vi "4155C Config QSCV var1 params.vi"(4 "Cap Step":dbl=0.1 min=0.0 max=10.0 format="%.2f", 5 "compliance":dbl=0.1 min=0.0 max=0.1 format="%^.2e", 6 "step":dbl=2.0 min=-100.0 max=100.0 format="%^.4e", 7 "sweep mode":u16(ring) items=["Single", "Double"], 8 "error in (no error)":errorcluster, 9 "stop":dbl=1.0 min=-100.0 max=100.0 format="%^.4e", 10 "start":dbl min=-100.0 max=100.0 format="%^.4e", 11 "VISA session":refnum<visa-resource-name>) -> (0 "error out":errorcluster, 2 "Number of points":i32=1, 3 "dup VISA resource name":refnum<visa-resource-name>)   [LabVIEW 2016]
doc: "This VI configures the primary sweep source (VAR1) for a sweep mode measurement. \n* This VI does not perform error checking on MEASUREMENT MODE or UNIT TYPE of VAR1, therefore it is the application programmer's responsibility to make certain this VI is used in the proper mode."
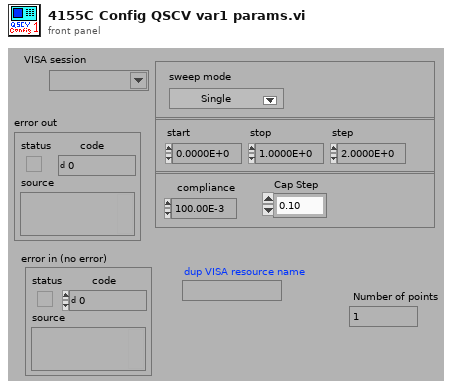
[diagram p1: front panel]
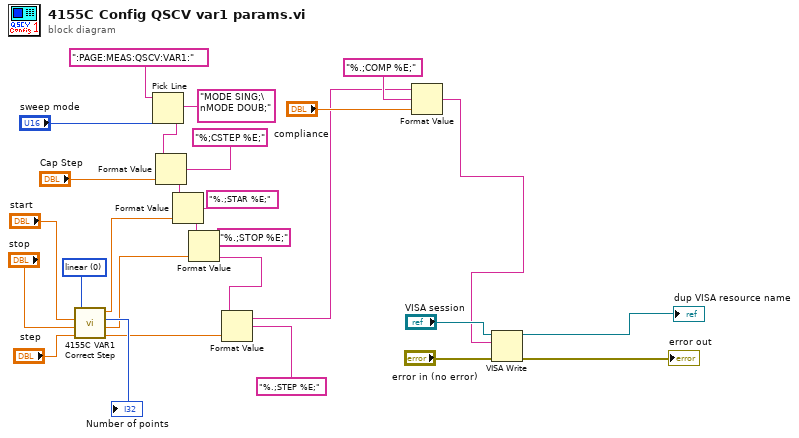
[diagram p0: block diagram]
diagram:
  w7 = u16 0 items=["linear", "log 10", "log 25", "log 50"] ("sweep spacing (linear: 0)")
  n1 = call "4155C VAR1 Correct Step.vi"("step"="step", "stop"="stop", "start"="start", "sweep spacing (linear: 0)"=w7) -> ("Corrected Step"=w4:dbl, "Corrected Stop"=w10:dbl, "Number of points"=→"Number of points":i32, "dup start"=w11:dbl)  [unwired: 4 in]
  n2 = Pick Line(string ("")=":PAGE:MEAS:QSCV:VAR1:", multi-line string="MODE SING;\nMODE DOUB;", line index="sweep mode") -> (output string=w18:string)
  n3 = Format Value(string ("")=w18, format string="%;CSTEP %E;", value (0)="Cap Step") -> (output string=w20:string)
  n4 = Format Value(string ("")=w20, format string="%.;STAR %E;", value (0)=w11) -> (output string=w26:string)
  n5 = Format Value(string ("")=w26, format string="%.;STOP %E;", value (0)=w10) -> (output string=w2:string)
  n6 = Format Value(string ("")=w2, format string="%.;STEP %E;", value (0)=w4) -> (output string=w1:string)
  n7 = Format Value(string ("")=w1, format string="%.;COMP %E;", value (0)="compliance") -> (output string=w5:string)
  n8 = VISA Write(VISA resource name="VISA session", write buffer=w5, error in (no error)="error in (no error)") -> (VISA resource name out=→"dup VISA resource name":refnum<visa-resource-name>, error out=→"error out":errorcluster)  [unwired: 1 out]
